vi "Merge.vi"(8 "Merge Threshold":dbl=200.0, 11 "Original Lines":T1[](array[typedef])) -> (3 "Merged Lines":T1[](array[typedef]))   [LabVIEW 2017]
uses:
  Vector Library/Line.ctl
  Vector Library/Vector.ctl
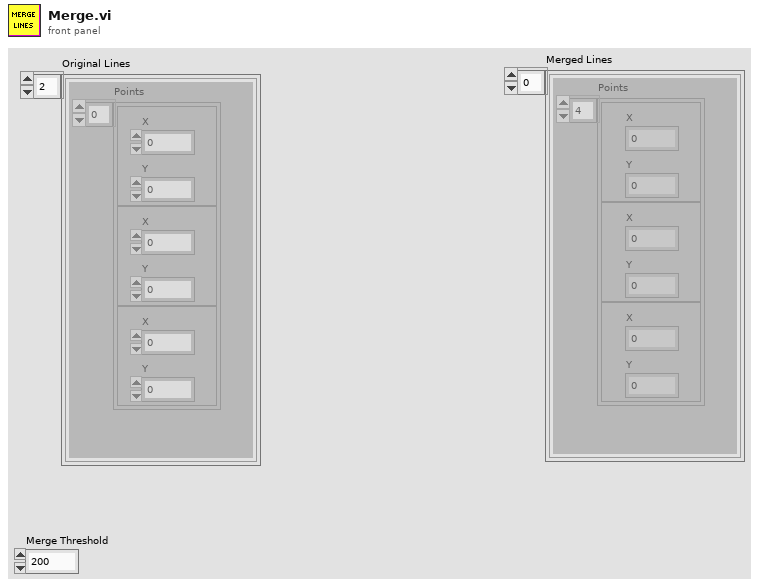
[diagram p1: front panel]
types:
  T1 = typedef "Line.ctl" = cluster{"Points":T2[]}
  T2 = typedef "Vector.ctl" = cluster{"X":dbl, "Y":dbl}
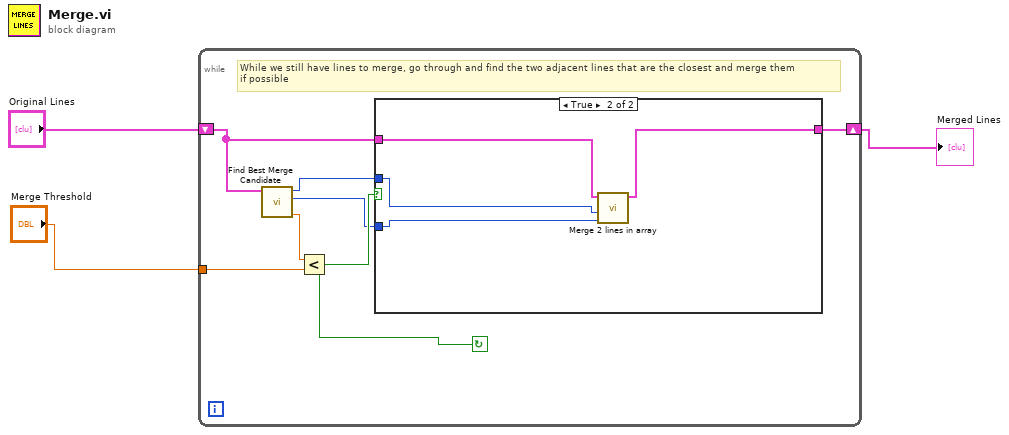
[diagram p0: block diagram]
diagram:
  n1 = while {
    shift-right: [w7] -> w1
    shift-left: "Original Lines" -> [w8]
    tunnel: "Merge Threshold" -> [w6]
    stop <- w10 continue-if-true
    # "While we still have lines to merge, go through and find the two adjacent lines that are the closest and merge them\nif possible"
    n2 = call "Find Best Merge Candidate.vi"("Lines"=w8) -> ("Best Match Outlier Distance"=w5:dbl, "Best match second index"=w4:i32, "Best match first index"=w9:i32)  [unwired: 8 in]
    n3 = Less?(x=w5, y=w6) -> (x < y?=w10:bool)
    n4 = case shown="True" w10 {
      tunnel: w9 -> [_ w13]
      tunnel: w8 -> [w11 w15]
      tunnel: [w11 w12] -> w7
      tunnel: w4 -> [_ w14]
      frame False {
      }
      frame True {
        n5 = call "Merge 2 lines in array.vi"("Index of 2nd line to merge"=w14, "Index of 1st line to merge"=w13, "Lines"=w15) -> ("Merged Lines"=w12:T1[])  [unwired: 8 in]
      }
    }
  }
  "Merged Lines" <- w1
